vi "Configure Math Function (Trend).vi"(4 "Math Function Index (1: Math Function 1)":i32(ring)=1 items=["Math Function 1"=1, "Math Function 2"=2, "Math Function 3"=3, "Math Function 4"=4], 8 "error in (no error)":errorcluster, 10 "Trend Measurement (4: Frequency)":i32(ring)=4 items=["Vaverage", "Acrms", "V Ratio", "Period", "Frequency", "Pwidth", "Nwidth", "Duty Cycle", "Rise Time", "Fall Time"], 11 "VISA resource name":refnum<visa-resource-name>) -> (0 "error out":errorcluster, 3 "VISA resource name out":refnum<visa-resource-name>)   [LabVIEW 2017, in "Agilent 2000 3000 X-Series.lvlib"]
doc: "Configures the trend math function.\n\n<B>Note(s):</B>\n1000, MSOX/DSOX 3000G series are not supported"
uses:
  Agilent 2000 3000 X-Series.lvlib
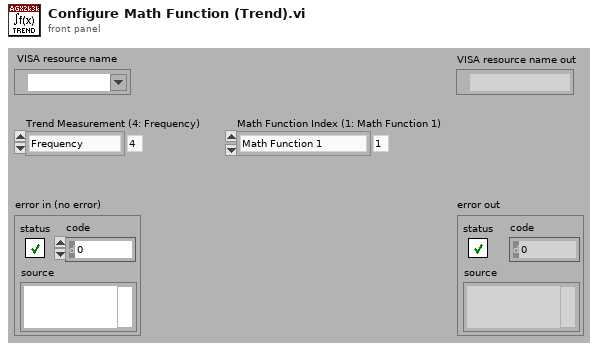
[diagram p1: front panel]
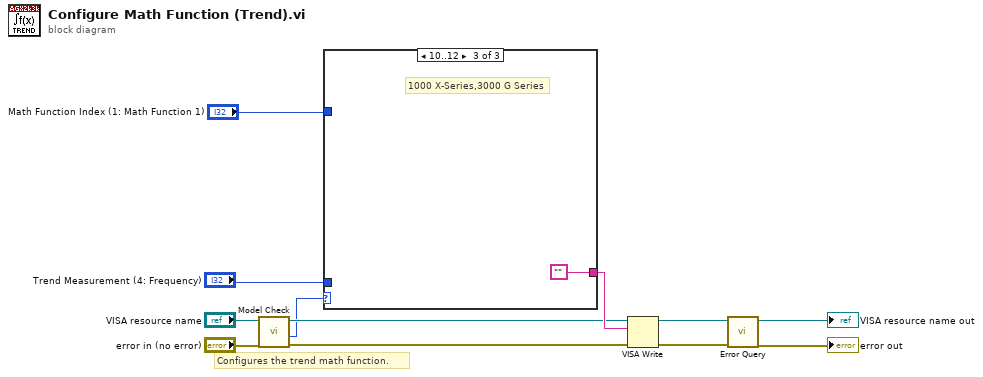
[diagram p0: block diagram]
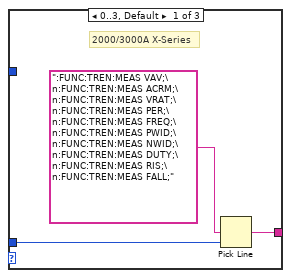
[diagram p2: hidden frame]
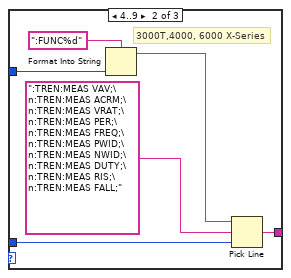
[diagram p3: hidden frame]
diagram:
  # "Configures the trend math function."
  n1 = call "Model Check.vi"("error in (no error)"="error in (no error)", "VISA resource name"="VISA resource name") -> ("error out"=w4:errorcluster, "Model"=w1:i32, "VISA resource name out"=w3:refnum<visa-resource-name>)  [unwired: 7 out]
  n2 = case shown="10..12" w1 {
    tunnel: "Trend Measurement (4: Frequency)" -> [w14 w19 _]
    tunnel: [w13 w20 ""] -> w11
    tunnel: "Math Function Index (1: Math Function 1)" -> [_ w17 _]
    frame 0..3, Default {
      # "2000/3000A X-Series"
      n3 = Pick Line(multi-line string=":FUNC:TREN:MEAS VAV;\n:FUNC:TREN:MEAS ACRM;\n:FUNC:TREN:MEAS VRAT;\n:FUNC:TREN:MEAS PER;\n:FUNC:TREN:MEAS FREQ;\n:FUNC:TREN:MEAS PWID;\n:FUNC:TREN:MEAS NWID;\n:FUNC:TREN:MEAS DUTY;\n:FUNC:TREN:MEAS RIS;\n:FUNC:TREN:MEAS FALL;", line index=w14) -> (output string=w13:string)  [unwired: 1 out]
    }
    frame 4..9 {
      # "3000T,4000, 6000 X-Series"
      n4 = Format Into String(format string=":FUNC%d", w17) -> (resulting string=w16:string)  [unwired: 2 in, 1 out]
      n5 = Pick Line(string ("")=w16, multi-line string=":TREN:MEAS VAV;\n:TREN:MEAS ACRM;\n:TREN:MEAS VRAT;\n:TREN:MEAS PER;\n:TREN:MEAS FREQ;\n:TREN:MEAS PWID;\n:TREN:MEAS NWID;\n:TREN:MEAS DUTY;\n:TREN:MEAS RIS;\n:TREN:MEAS FALL;", line index=w19) -> (output string=w20:string)
    }
    frame 10..12 {
      # "1000 X-Series,3000 G Series"
    }
  }
  n6 = VISA Write(VISA resource name=w3, write buffer=w11, error in (no error)=w4) -> (VISA resource name out=w10:refnum<visa-resource-name>, error out=w9:errorcluster)  [unwired: 1 out]
  n7 = call "Error Query.vi"("error in (no error)"=w9, "VISA resource name"=w10) -> ("error out"=→"error out":errorcluster, "VISA resource name out"=→"VISA resource name out":refnum<visa-resource-name>)  [unwired: 8 out]
